vi "Main.vi"(8 "error in (no error)":errorcluster) -> (0 "error out":errorcluster)   [LabVIEW 2022 SP3, in "TouchControl.lvlib" / "TouchControl.lvclass"]
uses:
  TouchControl.lvclass
  TouchControl.lvclass/TouchControl.ctl
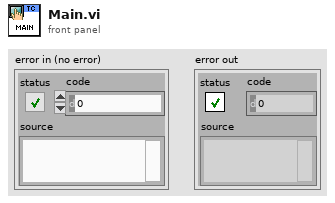
[diagram p1: front panel]
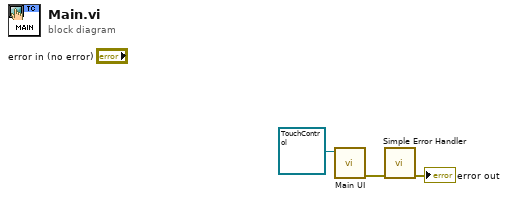
[diagram p0: block diagram]
diagram:
  n1 = call "Main UI.vi"("TouchControl in"=refnum<class "TouchControl.lvclass"> refnum) -> ("error out"=w2:errorcluster)  [unwired: 9 in, 1 out]
  n2 = call <vilib>:"Simple Error Handler.vi"("error in (no error)"=w2) -> ("error out"=→"error out":errorcluster)  [unwired: 4 in, 4 out]
